vi "Send Software Trigger.vi"(8 "error in (no error)":errorcluster, 11 "VISA resource name":refnum<visa-resource-name>) -> (0 "error out":errorcluster, 3 "VISA resource name out":refnum<visa-resource-name>)   [LabVIEW 2015, in "Agilent 34401.lvlib"]
doc: "This low-level VI sends a software bus trigger to the instrument. You can use software bus triggers to trigger multipoint measurements. You must first set Trigger Source to Software in the <B>Configure Trigger VI</B>, and specify the Trigger Count in the <B>Configure Multipoint VI</B>. After the call to <B>Initiate Measurement VI</B>, send the software bus triggers by calling this VI repeatedly. When triggers are complete, call the <B>Fetch Measurement VI</B> in a loop until completion.\n\n<B>Note:</B>\n\nThis VI does not check the instrument status. Typically, you call this VI only in a sequence of calls to other low-level instrument driver VIs. The sequence performs one operation. You use the low-level VIs to optimize one or more aspects of interaction with the instrument. If you want to check the instrument status, call the <B>Error Query VI</B> at the conclusion of the sequence."
uses:
  <instrlib>/Agilent 34401/Agilent 34401.lvlib
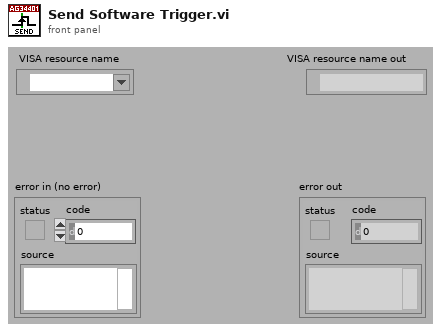
[diagram p1: front panel]
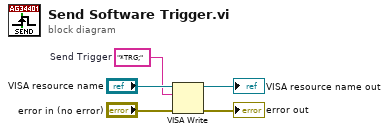
[diagram p0: block diagram]
diagram:
  w3 = "*TRG;"  # Send Trigger
  n1 = VISA Write(VISA resource name="VISA resource name", write buffer=w3, error in (no error)="error in (no error)") -> (VISA resource name out=→"VISA resource name out":refnum<visa-resource-name>, error out=→"error out":errorcluster)  [unwired: 1 out]
